vi "Get Collection Size.vi"(11 "PacketCollection in":refnum<class "PacketCollection.lvclass">) -> (2 "Collection size":i32, 3 "PacketCollection out":refnum<class "PacketCollection.lvclass">)   [LabVIEW 2013, in "MQTT Server.lvlib" / "PacketCollection.lvclass"]
uses:
  PacketCollection.lvclass
  PacketCollection.lvclass/PacketCollection.ctl
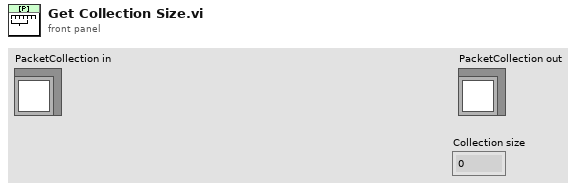
[diagram p1: front panel]
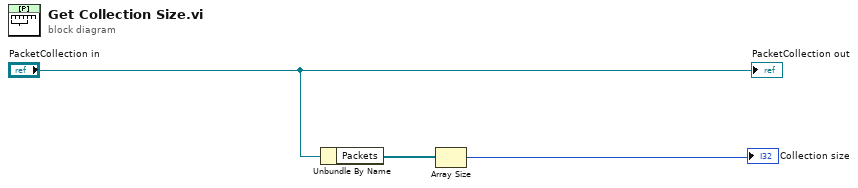
[diagram p0: block diagram]
diagram:
  n1 = Unbundle By Name("PacketCollection in") -> ("Packets"=w2:refnum<class "ControlPacket.lvclass">[])
  n2 = Array Size(array=w2) -> (size(s)=→"Collection size":i32)
  "PacketCollection out" <- "PacketCollection in"
